vi "get all classes in packed library.vi"(8 "error in":errorcluster, 11 "packed library path":path) -> (0 "error out":errorcluster, 2 "all class names[]":string[](array[string]), 3 "all classes path":path[](array[path]))   [LabVIEW 2023, in "Reusable Library.lvlib"]
uses:
  Reusable Library.lvlib
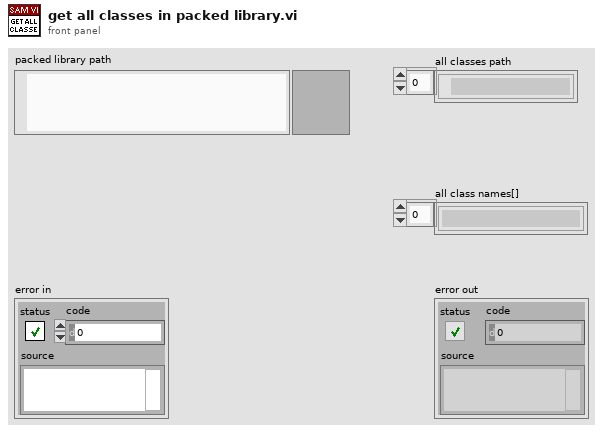
[diagram p1: front panel]
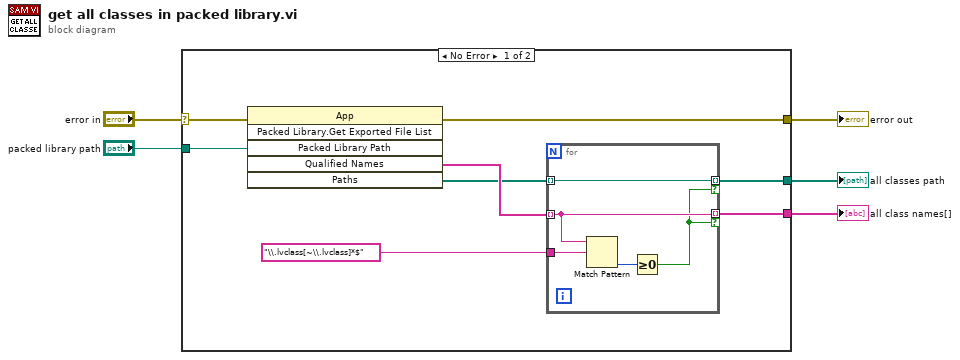
[diagram p0: block diagram]
diagram:
  n1 = case shown="No Error" "error in" {
    selector: "error in" -> [w12 w19]
    tunnel: "packed library path" -> [w13 _]
    tunnel: [w9 _] -> w3
    tunnel: [w7 _] -> w2
    tunnel: [w6 w19] -> w1
    frame No Error {
      n2 = invoke class="App" method="Packed Library.Get Exported File List"(error in=w12, "Packed Library Path"=w13) -> (error out=w6:errorcluster, "Qualified Names"=w10:string[], "Paths"=w8:path[])  [unwired: 4 in, 3 out]
      n3 = for {
        tunnel: "\\.lvclass[~\\.lvclass]*$" ("regular expression") -> [w18]
        tunnel: w10 -> [w15] mode=indexing
        tunnel: [w17] -> w9 mode=indexing if=w14
        tunnel: w8 -> [w17] mode=indexing
        tunnel: [w15] -> w7 mode=indexing if=w14
        n4 = Match Pattern(string=w15, regular expression=w18) -> (offset past match=w16:i32)  [unwired: 4 out]
        n5 = Greater Or Equal To 0?(x=w16) -> (x >= 0?=w14:bool)
      }
    }
    frame Error {
    }
  }
  "all classes path" <- w3
  "all class names[]" <- w2
  "error out" <- w1
